vi "excecuteCommand.vi"(6 "inputValue":sgl, 8 "error in (no error)":errorcluster, 9 "id":T3=1, 10 "CoolerCommand":T2, 11 "CoolerControler in":refnum<class "CoolerControler.lvclass">) -> (0 "error out":errorcluster, 2 "response out":T1, 3 "CoolerControler out":refnum<class "CoolerControler.lvclass">)   [LabVIEW 2016, in "CoolerControler.lvclass"]
uses:
  CoolerControler.lvclass
  typedefs/CoolerId.ctl
  typedefs/CoolerCommands.ctl
  typedefs/response.ctl
  SerialCommand/CoolerSerialCommand.lvclass
  CoolerControler.lvclass/CoolerControler.ctl
  common_serial_tcpextended/Communicator/Communicator.lvclass
panel:
  out "error out 2":errorcluster
  out "validChecksum":bool
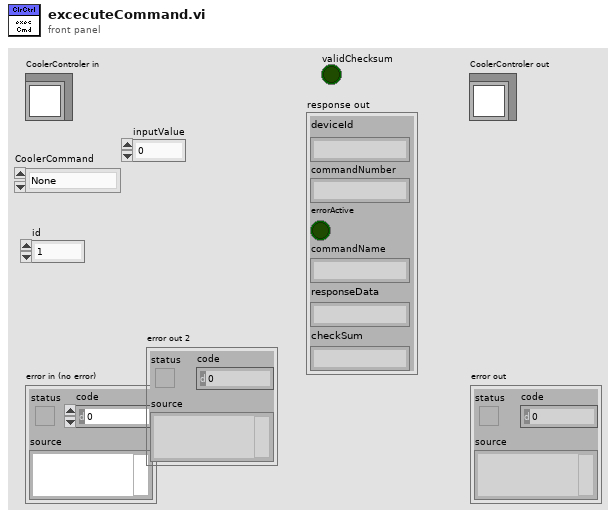
[diagram p1: front panel]
types:
  T1 = typedef "response.ctl" = cluster{"deviceId":string, "commandNumber":string, "errorActive":bool, "commandName":string, "responseData":string, "checkSum":string}
  T2 = typedef "CoolerCommands.ctl" = enum16{"None", "SetExternSensorStatus", "SetChillerStatus", "SetControlSensor", "SetControlTemperature", "SetHighSupplyTempWarning", "SetLowSupplyTemperatureWarning", "SetHighAmbientTemperatureWarning", "SetLowAmbienTemperatureWarning", "SetLowProcessFlowWarning", "SetHighSupplyTemperatureAlarm", "SetLowSupplyTemperatureAlarm", "SetHighAmbientTemperatureAlarm", "SetLowAmbientTemperatureAlarm", "SetLowProcessFlowAlarm"}
  T3 = typedef "CoolerId.ctl" = u16
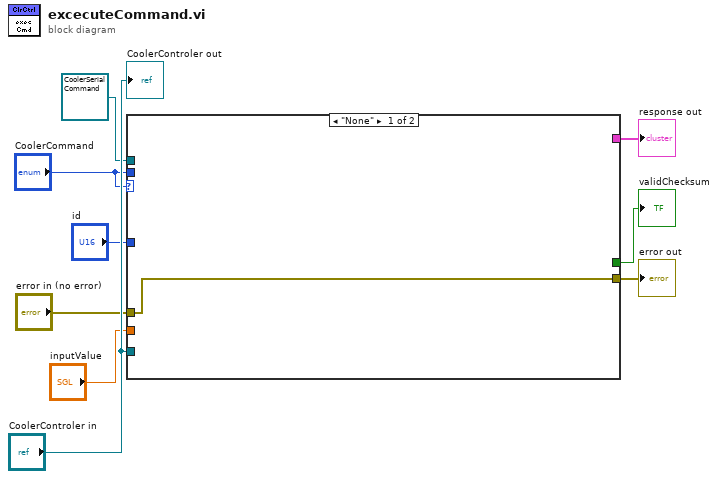
[diagram p0: block diagram]
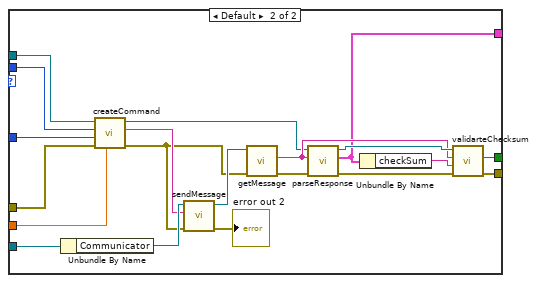
[diagram p2: hidden frame]
diagram:
  n1 = case shown="\"None\"" "CoolerCommand" {
    tunnel: [w10 w22] -> w9
    tunnel: [_ w21] -> w8
    tunnel: [_ w20] -> w7
    tunnel: "CoolerControler in" -> [_ w19]
    tunnel: "error in (no error)" -> [w10 w15]
    tunnel: "id" -> [_ w14]
    tunnel: "CoolerCommand" -> [_ w13]
    tunnel: refnum<class "CoolerSerialCommand.lvclass"> refnum ("CoolerSerialCommand.lvclass") -> [_ w12]
    tunnel: "inputValue" -> [_ w11]
    frame "None" {
    }
    frame Default {
      n2 = Unbundle By Name(w19) -> ("Communicator"=w30:refnum<class "Communicator.lvclass">)
      n3 = call "createCommand.vi"("inputValue"=w11, "error in (no error)"=w15, "id"=w14, "commands"=w13, "CoolerSerialCommand in"=w12) -> ("error out"=w16:errorcluster, "SerialCommandStr"=w17:string, "CoolerSerialCommand out"=w18:refnum<class "CoolerSerialCommand.lvclass">)  [unwired: 4 in]
      n4 = call-dynamic "sendMessage.vi"("error in (no error)"=w16, "message"=w17, "Communicator in"=w30) -> ("error out"=→"error out 2":errorcluster, "Communicator out"=w29:refnum<class "Communicator.lvclass">)  [unwired: 7 in]
      n5 = call-dynamic "getMessage.vi"("error in (no error)"=w16, "Communicator in"=w29) -> ("error out"=w28:errorcluster, "String"=w25:string)  [unwired: 7 in, 1 out]
      n6 = call "parseResponse.vi"("error in (no error)"=w28, "response in"=w25, "CoolerSerialCommand in"=w18) -> ("error out"=w26:errorcluster, "response out"=w20:T1, "CoolerSerialCommand out"=w27:refnum<class "CoolerSerialCommand.lvclass">)  [unwired: 6 in]
      n7 = Unbundle By Name(w20) -> ("checkSum"=w24:string)
      n8 = call "validarteChecksum.vi"("error in (no error)"=w26, "checkSum"=w24, "response"=w25, "CoolerSerialCommand in"=w27) -> ("error out"=w22:errorcluster, "validChecksum"=w21:bool)  [unwired: 5 in, 1 out]
    }
  }
  "error out" <- w9
  "response out" <- w7
  "validChecksum" <- w8
  "CoolerControler out" <- "CoolerControler in"
